vi "S2C_5190CR_Proc_Initialize.vi"(7 "Local?":bool, 8 "Error In":errorcluster, 10 "Command":string, 11 "JSON String":string) -> (0 "Error Out":errorcluster, 3 "Response":variant)   [LabVIEW 2015]
doc: "Initializes the 5190CR PDU equipment."
uses:
  S2C_5190CR_Proc_Globals.vi
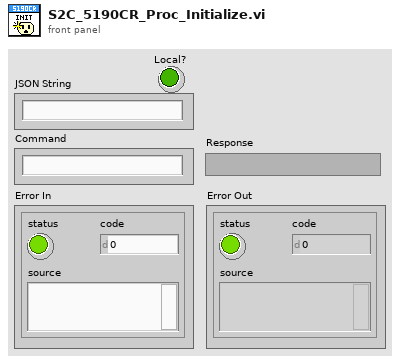
[diagram p1: front panel]
types:
  T1 = cluster{"IP Address":string, "Port":u16, "Username":string, "Password":string, "Timeout(ms)":i32}
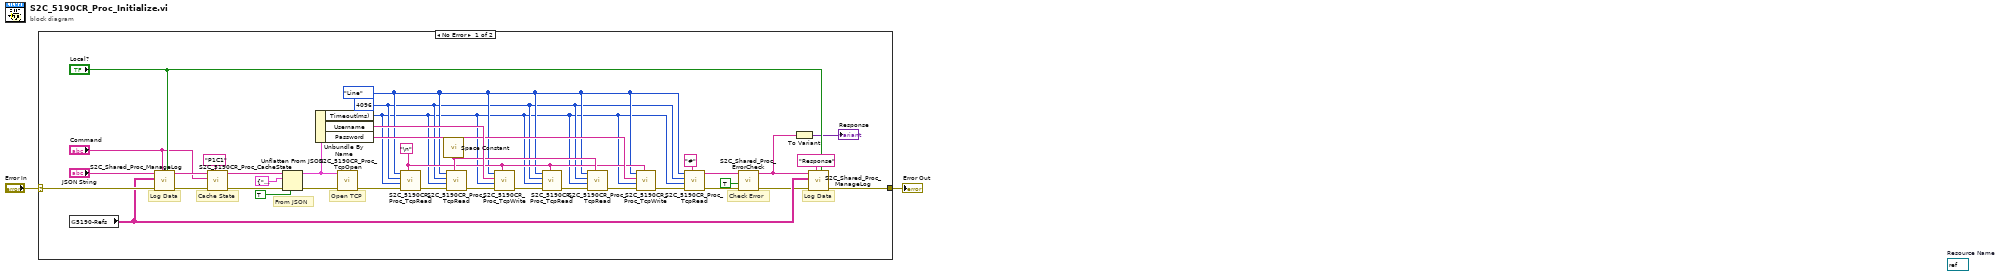
[diagram p0: block diagram]
diagram:
  (unwired) refnum<visa-resource-name> refnum  # Resource Name
  n1 = case shown="No Error" "Error In" {
    selector: "Error In" -> [w38 w40]
    tunnel: [w27 w40] -> w1
    frame No Error {
      w13 = "\n"
      w9 = enum16{"Normal", "Line"}."Line" ("Read Mode")
      w8 = 4096 ("Bytes")
      # "Check Error"
      # "Open TCP"
      # "Cache State"
      # "Log Data"
      # "Log Data"
      # "From JSON"
      n2 = global read "S2C_5190CR_Proc_Globals.vi" "5190-Refs"() -> (w26:string[][])
      n3 = call "S2C_Shared_Proc_ManageLog.vi"("Local?"="Local?", "Command"="Command", "Error In"=w38, "Refs"=w26, "Data In"="JSON String") -> ("Error Out"=w34:errorcluster, "Data Out"=w33:string)  [unwired: 5 in]
      n4 = call "S2C_5190CR_Proc_CacheState.vi"("Label"="P1C1", "Error In"=w34, "Command"="Command", "Data In"=w33) -> ("Error Out"=w31:errorcluster, "Data Out"=w32:string)  [unwired: 6 in]
      n5 = Unflatten From JSON(JSON string=w32, type and defaults=T1 {"IP Address"="", "Port"=57600, "Username"="", "Password"="", "Timeout(ms)"=5000} ("P1C1"), default null elements? (F)=TRUE, error in (no error)=w31) -> (value=w3:T1, error out=w29:errorcluster)  [unwired: 3 in]
      n6 = Unbundle By Name(w3) -> ("Timeout(ms)"=w7:i32, "Username"=w19:string, "Password"=w15:string)
      n7 = call "S2C_5190CR_Proc_TcpOpen.vi"("Error In"=w29, "Settings In"=w3) -> ("Error Out"=w28:errorcluster)  [unwired: 7 in, 2 out]
      n8 = call "S2C_5190CR_Proc_TcpRead.vi"("Line Seperator"=w13, "Error In"=w28, "Timeout(ms)"=w7, "Bytes"=w8, "Read Mode"=w9) -> ("Error Out"=w21:errorcluster)  [unwired: 5 in, 1 out]
      n9 = call <vilib>:"Space Constant.vi"() -> ("String"=w14:string)
      n10 = call "S2C_5190CR_Proc_TcpRead.vi"("Line Seperator"=w14, "Error In"=w21, "Timeout(ms)"=w7, "Bytes"=w8, "Read Mode"=w9) -> ("Error Out"=w20:errorcluster)  [unwired: 5 in, 1 out]
      n11 = call "S2C_5190CR_Proc_TcpWrite.vi"("Line Seperator"=w13, "Error In"=w20, "Timeout(ms)"=w7, "Data"=w19, "Write Mode"=w9) -> ("Error Out"=w16:errorcluster)  [unwired: 6 in]
      n12 = call "S2C_5190CR_Proc_TcpRead.vi"("Line Seperator"=w13, "Error In"=w16, "Timeout(ms)"=w7, "Bytes"=w8, "Read Mode"=w9) -> ("Error Out"=w17:errorcluster)  [unwired: 5 in, 1 out]
      n13 = call "S2C_5190CR_Proc_TcpRead.vi"("Line Seperator"=w14, "Error In"=w17, "Timeout(ms)"=w7, "Bytes"=w8, "Read Mode"=w9) -> ("Error Out"=w18:errorcluster)  [unwired: 5 in, 1 out]
      n14 = call "S2C_5190CR_Proc_TcpWrite.vi"("Line Seperator"=w13, "Error In"=w18, "Timeout(ms)"=w7, "Data"=w15, "Write Mode"=w9) -> ("Error Out"=w10:errorcluster)  [unwired: 6 in]
      n15 = call "S2C_5190CR_Proc_TcpRead.vi"("Line Seperator"="#", "Error In"=w10, "Timeout(ms)"=w7, "Bytes"=w8, "Read Mode"=w9) -> ("Error Out"=w12:errorcluster, "Data"=w11:string)  [unwired: 5 in]
      n16 = call "S2C_Shared_Proc_ErrorCheck.vi"("Error In"=w12, "ExpReply?"=TRUE, "Reply Text"=w11) -> ("Error Out"=w25:errorcluster, "Status"=w24:string)  [unwired: 7 in]
      n17 = To Variant(anything=w24) -> (Variant=→"Response":variant)
      n18 = call "S2C_Shared_Proc_ManageLog.vi"("Local?"="Local?", "Command"="Response", "Error In"=w25, "Refs"=w26, "Data In"=w24) -> ("Error Out"=w27:errorcluster)  [unwired: 5 in, 1 out]
    }
    frame Error {
    }
  }
  "Error Out" <- w1
